vi "Parse CSM Log LIne.vi"(11 "LogString":string) -> (3 "cluster":T1 {"Timestamp" format="%<%.3X %x>T"})   [LabVIEW 2020]
uses:
  Typedef/Def - Parsed CSMLog Line - Cluster.ctl
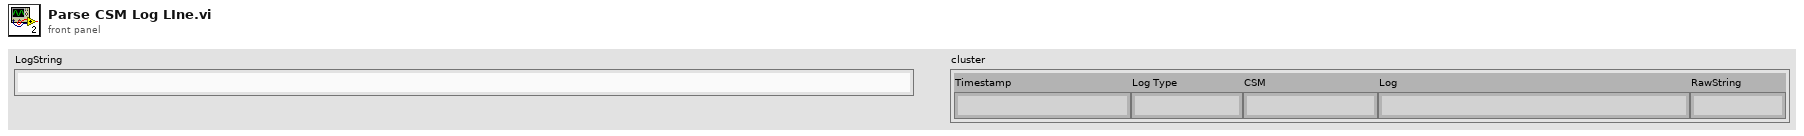
[diagram p1: front panel]
types:
  T1 = typedef "Def - Parsed CSMLog Line - Cluster.ctl" = cluster{"Timestamp":timestamp, "Log Type":string, "CSM":string, "Log":string, "RawString":string}
  T2 = cluster{timestamp, "LogString":string, "LogString":string, "LogString":string, "LogString":string}
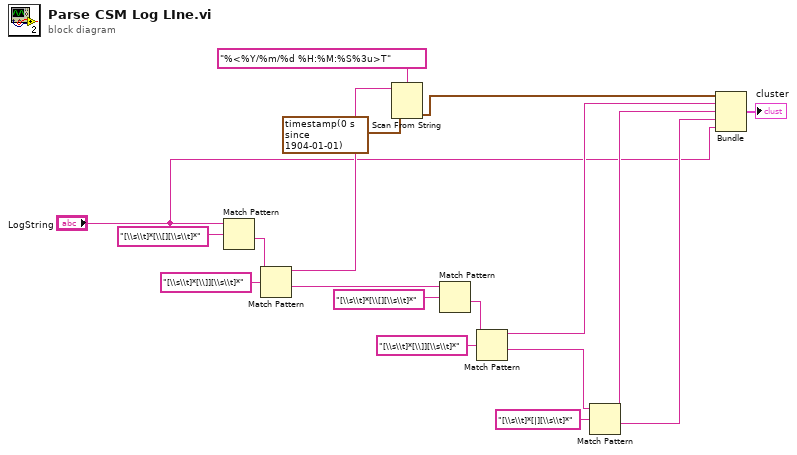
[diagram p0: block diagram]
diagram:
  n1 = Match Pattern(string="LogString", regular expression="[\\s\\t]*[\\[][\\s\\t]*") -> (after substring=w17:string)  [unwired: 1 in, 3 out]
  n2 = Match Pattern(string=w17, regular expression="[\\s\\t]*[\\]][\\s\\t]*") -> (before substring=w15:string, after substring=w9:string)  [unwired: 1 in, 2 out]
  n3 = Scan From String(format string="%<%Y/%m/%d %H:%M:%S%3u>T", input string=w15, default 1=timestamp(0 s since 1904-01-01)) -> (output 1=w8:timestamp)  [unwired: 2 in, 3 out]
  n4 = Match Pattern(string=w9, regular expression="[\\s\\t]*[\\[][\\s\\t]*") -> (after substring=w11:string)  [unwired: 1 in, 3 out]
  n5 = Match Pattern(string=w11, regular expression="[\\s\\t]*[\\]][\\s\\t]*") -> (before substring=w6:string, after substring=w1:string)  [unwired: 1 in, 2 out]
  n6 = Match Pattern(string=w1, regular expression="[\\s\\t]*[|][\\s\\t]*") -> (before substring=w5:string, after substring=w4:string)  [unwired: 1 in, 2 out]
  n7 = Bundle(w8, "LogString"=w6, "LogString"=w5, "LogString"=w4, "LogString"="LogString") -> (→"cluster":T2)  [unwired: 1 in]
